vi "is module registered.vi"(8 "error in":errorcluster, 10 "module ID":string, 11 "engine configuration in":refnum<class "engine configuration.lvclass">) -> (0 "error out":errorcluster, 2 "registered?":bool, 3 "engine configuration out":refnum<class "engine configuration.lvclass">)   [LabVIEW 2013, in "engine configuration.lvclass"]
doc: "This function returns whether or not a given module has been registered with the engine."
uses:
  engine configuration.lvclass
  engine configuration.lvclass/engine configuration.ctl
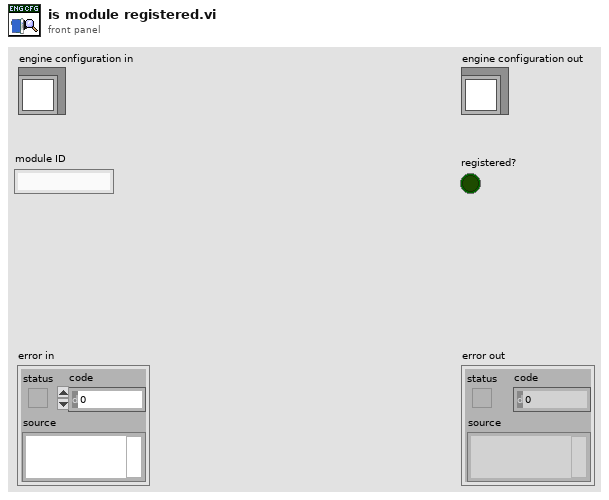
[diagram p1: front panel]
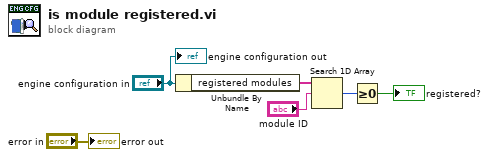
[diagram p0: block diagram]
diagram:
  n1 = Unbundle By Name("engine configuration in") -> ("registered modules"=w3:string[])
  n2 = Search 1D Array(1D array=w3, element="module ID") -> (index of element=w2:i32)  [unwired: 1 in]
  n3 = Greater Or Equal To 0?(x=w2) -> (x >= 0?=→"registered?":bool)
  "error out" <- "error in"
  "engine configuration out" <- "engine configuration in"
